vi "Find Bad Pointers.vi"(7 "Unique ID":string, 8 "error in (no error)":errorcluster, 10 "Removed Unique ID":string, 11 "Linked List in":refnum<class "Linked List.lvclass">) -> (0 "error out":errorcluster, 2 "Bad Pointers":string[](array[string]), 3 "Linked List out":refnum<class "Linked List.lvclass">)   [LabVIEW 2020, in "Linked Lists.lvlib" / "Linked List.lvclass"]
uses:
  <vilib>/gpm_packages/@cs/linked-list/Source/Linked List/Linked List/Linked List.lvclass
  <vilib>/gpm_packages/@cs/linked-list/Source/Linked List/Linked List Definition/Linked List Definition.lvclass
  <vilib>/gpm_packages/@cs/linked-list/Source/Linked List/Linked List/Linked List.lvclass/Linked List.ctl
  <vilib>/gpm_packages/@cs/lookup-table/Source/LookupTable/LookupTable.lvclass/LookupTable.ctl
  411249fd-342a-49a8-9fce-24532ec06efa.vi
  d8d1c3c1-ee0d-437f-98f0-79b0e53df3ec.vi
  <vilib>/gpm_packages/@cs/lookup-table/Source/LookupTable/Read Table Reference.vi
  411249fd-342a-49a8-9fce-24532ec06efa.vi/5a7267ad-595e-4610-9ac2-8bef780848ff.vi
  d8d1c3c1-ee0d-437f-98f0-79b0e53df3ec.vi/5a7267ad-595e-4610-9ac2-8bef780848ff.vi
  <vilib>/gpm_packages/@cs/lookup-table/Source/LookupTable/LookupTable.lvclass
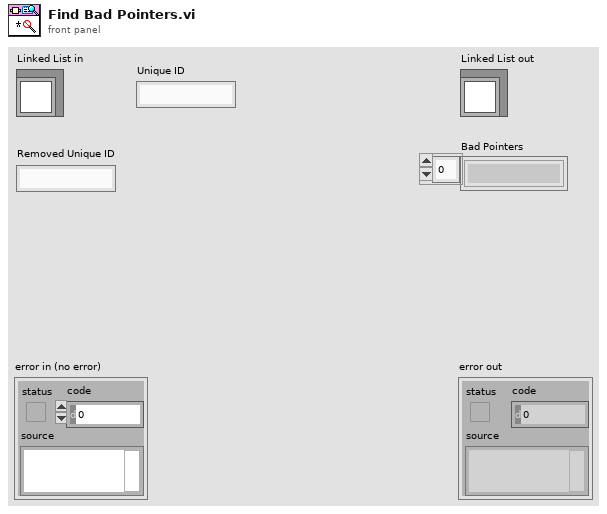
[diagram p1: front panel]
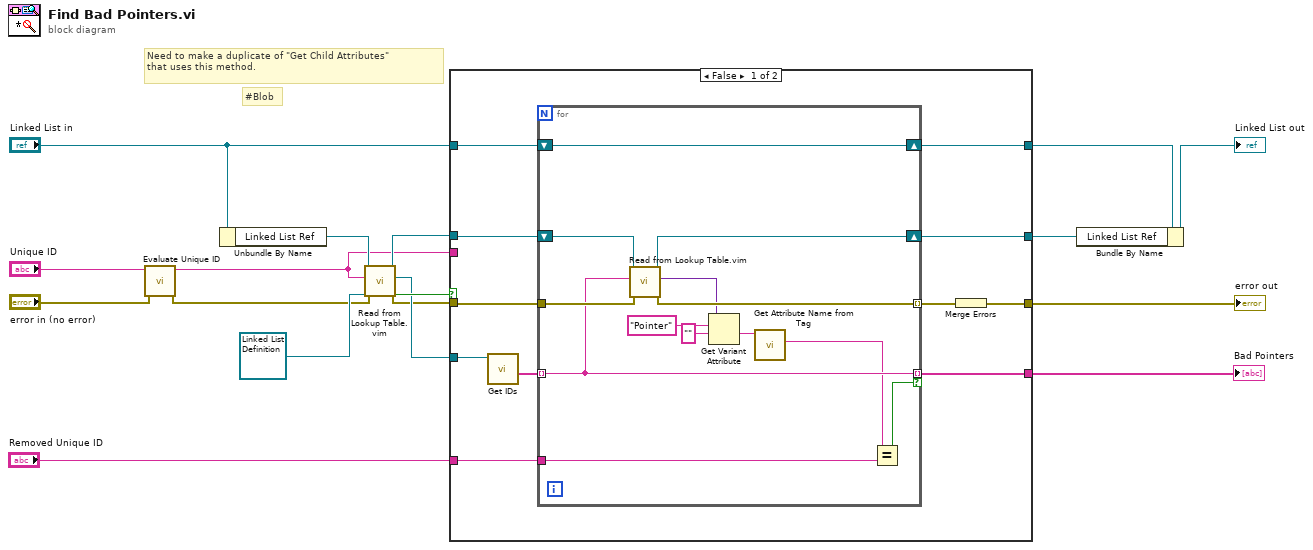
[diagram p0: block diagram]
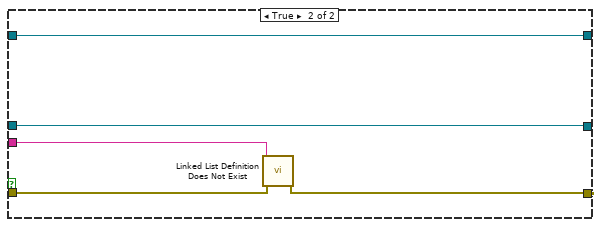
[diagram p2: hidden frame]
diagram:
  # "#Blob"
  # "Need to make a duplicate of \"Get Child Attributes\"\nthat uses this method."
  n1 = call <vilib>:"Evaluate Unique ID.vi"("error in (no error)"="error in (no error)", "Unique ID"="Unique ID") -> ("error out"=w13:errorcluster, "Unique ID Out"=w10:string)  [unwired: 8 in]
  n2 = Unbundle By Name("Linked List in") -> ("Linked List Ref"=w15:refnum<data-value>)
  n3 = call "Read from Lookup Table.vim"("error in (no error)"=w13, "Type"=refnum<class "Linked List Definition.lvclass"> refnum ("Linked List.lvlib:Linked List Definition.lvclass"), "Item Name"=w10, "LookupTable Reference"=w15) -> ("error out"=w8:errorcluster, "Not Found?"=w12:bool, "Value"=w9:refnum<class "Linked List Definition.lvclass">, "LookupTable Reference Out"=w11:refnum<data-value>)  [unwired: 4 in]
  n4 = case shown="False" w12 {
    tunnel: w11 -> [w25 w42]
    tunnel: w10 -> [_ w45]
    tunnel: w9 -> [w23 _]
    tunnel: w8 -> [w24 w46]
    tunnel: [w26 w43] -> w3
    tunnel: "Linked List in" -> [w27 w43]
    tunnel: "Removed Unique ID" -> [w22 _]
    tunnel: [w20 w44] -> w2
    tunnel: [w19 w42] -> w5
    tunnel: [w18 _] -> w1
    frame False {
      n5 = call <vilib>:"Get IDs.vi"("Linked List Definition in"=w23) -> ("Data IDs"=w28:string[])  [unwired: 8 in, 2 out]
      n6 = for {
        shift-right: [w39] -> w19
        shift-left: w25 -> [w40]
        tunnel: w28 -> [w33] mode=indexing
        shift-right: [w36] -> w26
        shift-left: w27 -> [w36]
        tunnel: w24 -> [w41]
        tunnel: [w35] -> w21 mode=indexing
        tunnel: w22 -> [w34]
        tunnel: [w33] -> w18 mode=indexing if=w29
        n7 = call "Read from Lookup Table.vim"("error in (no error)"=w41, "Item Name"=w33, "LookupTable Reference"=w40) -> ("error out"=w35:errorcluster, "Value"=w30:variant, "LookupTable Reference Out"=w39:refnum<data-value>)  [unwired: 5 in, 1 out]
        n8 = Get Variant Attribute(Variant=w30, name="Pointer", default value (empty Variant)="") -> (value=w32:string)  [unwired: 1 in, 3 out]
        n9 = call <vilib>:"Get Attribute Name from Tag.vi"("Tag"=w32) -> ("Linked List ID"=w31:string)  [unwired: 8 in, 2 out]
        n10 = Equal?(x=w31, y=w34) -> (x = y?=w29:bool)
      }
      n11 = Merge Errors(w21) -> (w20:errorcluster)
    }
    frame True {
      n12 = call <vilib>:"Linked List Definition Does Not Exist.vi"("Error In"=w46, "Unique ID"=w45) -> ("Error Out"=w44:errorcluster)  [unwired: 9 in]
    }
  }
  "error out" <- w2
  "Bad Pointers" <- w1
  n13 = Bundle By Name(cluster=w3, "Linked List Ref"=w5) -> (→"Linked List out":refnum<class "Linked List.lvclass">)
